vi "Prompt Convert 1.0 - 1.4 to 1.7.vi"(1 "Prompt 1.0 - 1.4 Test Parameters":T2) -> (0 "Prompt 1.7 Test Parameters":T1)   [LabVIEW 2011]
uses:
  TypeDefs/Prompt Test Parameters v1.0-1.4.ctl
  TypeDefs/Prompt Test Parameters v1.7.ctl
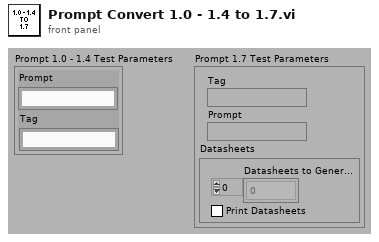
[diagram p1: front panel]
types:
  T1 = typedef "Prompt Test Parameters v1.7.ctl" = cluster{"Tag":string, "Prompt":string, "Datasheets":cluster{"Datasheets to Generate":i32[], "Print Datasheets":bool}}
  T2 = typedef "Prompt Test Parameters v1.0-1.4.ctl" = cluster{"Prompt":string, "Tag":string}
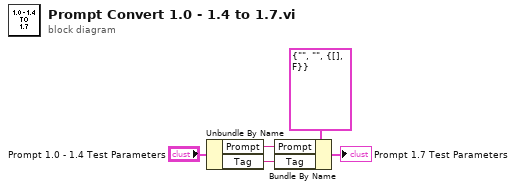
[diagram p0: block diagram]
diagram:
  n1 = Unbundle By Name("Prompt 1.0 - 1.4 Test Parameters") -> ("Prompt"=w5:string, "Tag"=w4:string)
  n2 = Bundle By Name(cluster=T1 {"Tag"="", "Prompt"="", "Datasheets"={"Datasheets to Generate"=[], "Print Datasheets"=FALSE}} ("Prompt Test Parameters"), "Prompt"=w5, "Tag"=w4) -> (→"Prompt 1.7 Test Parameters":T1)
